vi "Stop Init.vi"(8 "error in":errorcluster, 11 "SCADA in":refnum<class "EMS.lvclass">) -> (0 "error out":errorcluster, 3 "SCADA out":refnum<class "EMS.lvclass">)   [LabVIEW 2018, in "EMS Core.lvlib" / "EMS.lvclass"]
uses:
  EMS.lvclass
  C:/Program Files (x86)/National Instruments/LabVIEW 2018/vi.lib/ActorFramework/Actor/Actor.lvclass
  Controls/Microgrid State.ctl
  EMS.lvclass/EMS.ctl
  <vilib>/ActorFramework/Actor/Actor.lvclass/Actor.ctl
  <vilib>/ActorFramework/Message Enqueuer/Message Enqueuer.lvclass/Message Enqueuer.ctl
  EMS Messages/Return Microgrid State Msg/Return Microgrid State Msg.lvclass/Return Microgrid State Msg.ctl
  <vilib>/ActorFramework/Message Enqueuer/Init from Existing Queue.vi
  <vilib>/ActorFramework/Message Enqueuer/Enqueue.vi
  <vilib>/ActorFramework/Stop Msg/Stop Msg.lvclass
  C:/Program Files (x86)/National Instruments/LabVIEW 2018/vi.lib/ActorFramework/Message/Message.lvclass
  EMS Messages/Return Microgrid State Msg/Return Microgrid State Msg.lvclass
  EMS Messages/Device Discovery Init Msg/Device Discovery Init Msg.lvclass
  <vilib>/ActorFramework/Message Priority Queue/Priority Enqueue.vi
  <vilib>/ActorFramework/Message Enqueuer/Message Enqueuer.lvclass
  <vilib>/ActorFramework/Actor/Actor.lvclass
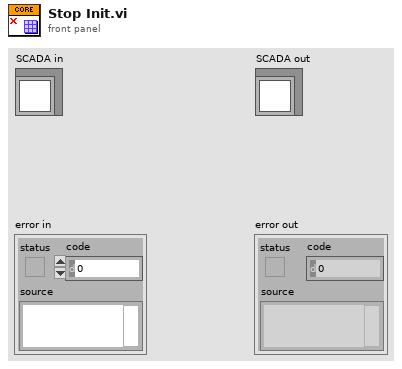
[diagram p1: front panel]
types:
  T1 = typedef "EMS Core.lvlib/EMS.lvclass/Microgrid State.ctl" = enum16{"Discovery", "Commissioning", "Activation", "Blackstart", "OnGrid", "OffGrid", "Island", "Resynchronization", "Manual", "Shutdown", "Stop"}
  T2 = typedef "EMS Core.lvlib/EMS.lvclass/IED Enqueuers.ctl" = cluster{"PV":refnum<class "Message Enqueuer.lvclass">, "IED":refnum<class "Message Enqueuer.lvclass">, "DER":refnum<class "Message Enqueuer.lvclass">, "Relay":refnum<class "Message Enqueuer.lvclass">, "PCC":refnum<class "Message Enqueuer.lvclass">, "ES":refnum<class "Message Enqueuer.lvclass">, "SmartRelay":refnum<class "Message Enqueuer.lvclass">, "ForecastData":refnum<class "Message Enqueuer.lvclass">, "PriceData":refnum<class "Message Enqueuer.lvclass">, "Load":refnum<class "Message Enqueuer.lvclass">, "HVAC":refnum<class "Message Enqueuer.lvclass">, "Meter":refnum<class "Message Enqueuer.lvclass">, "Generator":refnum<class "Message Enqueuer.lvclass">}
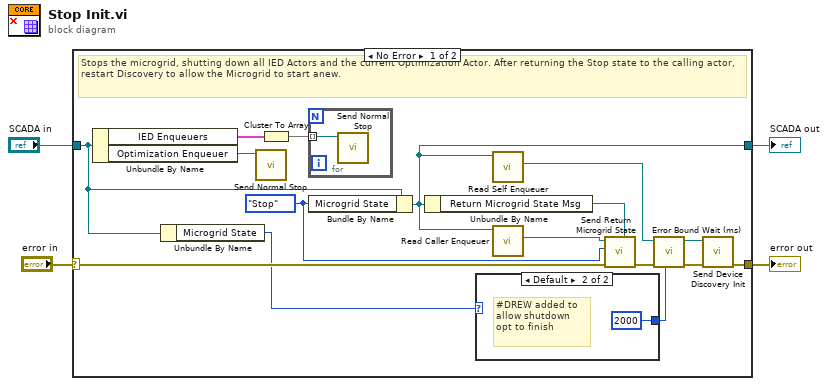
[diagram p0: block diagram]
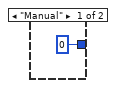
[diagram p2: hidden frame]
diagram:
  n1 = case shown="No Error" "error in" {
    selector: "error in" -> [w13 w24]
    tunnel: [w9 w24] -> w3
    tunnel: [w12 w23] -> w1
    tunnel: "SCADA in" -> [w6 w23]
    frame No Error {
      w17 = Microgrid_State."Stop" ("Microgrid State")
      # "Stops the microgrid, shutting down all IED Actors and the current Optimization Actor. After returning the Stop state to the calling actor, restart Discovery to allow the Microgrid to start anew."
      n2 = Unbundle By Name(w6) -> ("IED Enqueuers"=w16:T2, "Optimization Enqueuer"=w14:refnum<class "Message Enqueuer.lvclass">)
      n3 = Unbundle By Name(w6) -> ("Microgrid State"=w5:T1)
      n4 = call <vilib>:"Send Normal Stop.vi"("Message Enqueuer"=w14) -> ()  [unwired: 10 in, 1 out]
      n5 = Cluster To Array(cluster=w16) -> (array=w15:refnum<class "Message Enqueuer.lvclass">[])
      n6 = for {
        tunnel: w15 -> [w22] mode=indexing
        n7 = call <vilib>:"Send Normal Stop.vi"("Message Enqueuer"=w22) -> ()  [unwired: 10 in, 1 out]
      }
      n8 = Bundle By Name(cluster=w6, "Microgrid State"=w17) -> (w12:refnum<class "EMS.lvclass">)
      n9 = Unbundle By Name(w12) -> ("Return Microgrid State Msg"=w18:refnum<class "Return Microgrid State Msg.lvclass">)
      n10 = case shown="Default" w5 {
        tunnel: [u32 0 ("milliseconds to wait") u32 2000 ("milliseconds to wait")] -> w7
        frame "Manual" {
        }
        frame Default {
          # "#DREW added to allow shutdown opt to finish"
        }
      }
      n11 = call <vilib>:"Read Self Enqueuer.vi"("Actor"=w12) -> ("Self Enqueuer"=w11:refnum<class "Message Enqueuer.lvclass">)  [unwired: 10 in]
      n12 = call <vilib>:"Read Caller Enqueuer.vi"("Actor"=w12) -> ("Caller Enqueuer"=w19:refnum<class "Message Enqueuer.lvclass">)  [unwired: 10 in]
      n13 = call "Send Return Microgrid State.vi"("Message Type"=w18, "error in (no error)"=w13, "Microgrid State"=w17, "Message Enqueuer"=w19) -> ("error out"=w10:errorcluster)  [unwired: 6 in, 1 out]
      n14 = call "Error Bound Wait (ms).vi"("milliseconds to wait (100)"=w7, "error in"=w10) -> ("error out"=w8:errorcluster)  [unwired: 9 in]
      n15 = call "Send Device Discovery Init.vi"("error in (no error)"=w8, "Message Enqueuer"=w11) -> ("error out"=w9:errorcluster)  [unwired: 8 in, 1 out]
    }
    frame Error {
    }
  }
  "error out" <- w3
  "SCADA out" <- w1
